vi "Regenerate Hawkeye Files.vi"() -> ()   [LabVIEW 2019, in "HawkeyeToolsMenu.lvlib"]
doc: "GUI to compare LabVIEW code between currently checked out branch with any other branch or any of its commits.\n\n(c) 2024 Soliton Technologies. All rights reserved."
uses:
  HawkeyeToolsMenu.lvlib
  <vilib>/Hampel Software Engineering/Git API/Git API/GIT-api.lvclass
  <vilib>/Hampel Software Engineering/Git API/Git API/GIT-api.lvclass/GIT-api.ctl
  <vilib>/Hampel Software Engineering/Git API/Git API/Controls/GIT-Repository States.ctl
  <vilib>/Hampel Software Engineering/Git API/Git API/Accessors/GIT-Set Working Dir.vi
  <userlib>/_OpenG.lib/file/file.llb/File Exists - Scalar__ogtk.vi
  <userlib>/_OpenG.lib/file/file.llb/Valid Path - Traditional__ogtk.vi
  vi.lib/Hawkeye/Hawkeye.lvlib
panel:
  in  "Tab Control":T1(tab)=enum."Main UI"
  in  "LVLib / LVClass / Sub Folder Path":path
  out "Status Indicator":string
  in  "Check Changed Libraries Only?":bool
  in  "Branch to Compare":string(combo)
  in  "Refresh Current Branch":bool
  out "Current Branch":string="origin/main"
  out "Current Branch Status":string
  in  "Stop":bool
  in  "Repo / Workspace Folder Path":path
  in  "Generate":bool
  # "1. Checkout the branch of interest in your system using any method - Git command line, Desktop Git GUI Clients etc.,\n\n2. Specify the local Repository Path.\n\n3. Verify the current branch, its status and select a branch or commit based on the Compare Mode and click on Compare to display the file changes.\n\n4. Double click on a file to initiate LabVIEW code comparison.\n\n5. Once done with required comparisons, exit the tool by closing the window. The tool cleans up the temporary files added during comparison.\n\n\nNote:\n1. This tool uses LabVIEW's VI Comparison Tool which requires LabVIEW Professional Development System.\n2. It is recommended to not use other Git Clients actively when comparing files using this tool to avoid Git command related errors.\n3. It is recommended to commit all changes (working copy) before using this tool for comparison."
  # "This tool uses git diff command to identify the changes. Hence it is recommended to commit all the changes (working copy) to have them considered for comparison. For code comparison, this tool uses LabVIEW's built in VI Comparison Tool.\n\nExample: Identify changes in current branch when comparing with other branch\n\n---A---B---C---D    <== other branch\n               \\\n                 E---F      <== current branch\n\n1. We will need to identify only the file changes introduced by current branch. E and F commits are those changes in the above example (commits after the common ancestor B).\n2. For the identified file changes compare with the other branch (D) to see how it differs. These differences will be our current branch changelist.\n\nWhy only current branch changes?\nIt is most useful to see how the current branch will modify the files when it is getting merged. Best use case for displaying only current branch changelist will be for Pull Request reviews."
  # "1. Repository Path - Local repository path (the top level folder with '.git' hidden folder in it). Git API will be initialized for this repository.\n\n2. Current Branch - Currently checked out branch. The status of the current branch is also displayed at top right. Click Refresh button to update the current branch if it is changed in the system or received new changes via Git Pull.\n\n3. Compare Mode - Select the type of comparison. You can compare the current branch with another branch or with a particular commit of a selected branch.\n\nIn branch comparison mode, you can enter the branch name for comparison in Branch to Compare. Remote branches usually start with \"origin/\" and local branches do not have \"origin/\" prefix. The branch's recent commit is displayed in Recent Commit and its details in Commit Details for reference. \n\nIn commit comparison mode, the commits available in the branch selected in Select Branch are listed in Commit to Compare. For the commit selected in Commit to Compare, its details will be displayed in the Commit Details. Use Commits to Fetch to limit the number of commits obtained and improve the loading time.\n\n     Note: Git doesn't maintain information on when the branch is created. So, all the commits of the selected branch will be displayed (all the way up to the very first commit after repository creation). Without a limit, it increases loading time.\n\n4. Compare - Identifies the file changes and Current Branch Changelist table shows the list of all files that are different in the current branch compared to the branch/commit selected.\n\n     Note: The other branch/commit in comparison would have introduced its own changes that are not part of current branch. Those changes will not be displayed.\n\n5. Filter LabVIEW VI and Control Files - Filter files except VI and CTL files. These require LabVIEW to compare but project, library and classes are text files that can be easily reviewed in the desktop Git GUI clients or in Pull Request of Git web services.\n\n6. LabVIEW Compare Options - Options to decide what to compare in the code. Set the required options before initiating code compare.\n\n7. Double click on the file you wish to compare. LabVIEW opens the compare window for the file from the current branch and the file from the other branch/commit (file will be suffixed with TEMP). It may take a while if the VI/CTL have lot of dependencies to load. Having the project pre-opened and opening this tool from that instance may reduce the loading time. Note that the file from the other branch/commit in comparison may be missing its dependent files which may not be available in the current branch or deleted in the current branch commits. This will cause the file to be in a broken state but does not affect the comparison. Another reason for the broken state may be due to the parent library/class not recognizing this new file with the suffix but this as well will not affect the comparison.\n\n     Note: The files from other branch/commit are placed at the same location in the current branch so that the LabVIEW can load the dependencies appropriately.\n\n8. Viewed Status (mixed checkbox) - A tick mark appears for every file compared or opened. Use the mixed checkbox (below the Current Branch Changelist) to control status for all files.\n\n     Note: Viewed status is only a visual aid for tracking and does not have any other function other than that.\n\n9. Panel Close - Stops the tools execution after removing all the new files introduced into the current branch (TEMP files)."
  # "This GUI helps identify unexpected dependencies across all libraries in a repository. It also supports branch-to-branch comparison, allowing users to analyze dependency changes between any two branches and validate dependencies only for the modified libraries."
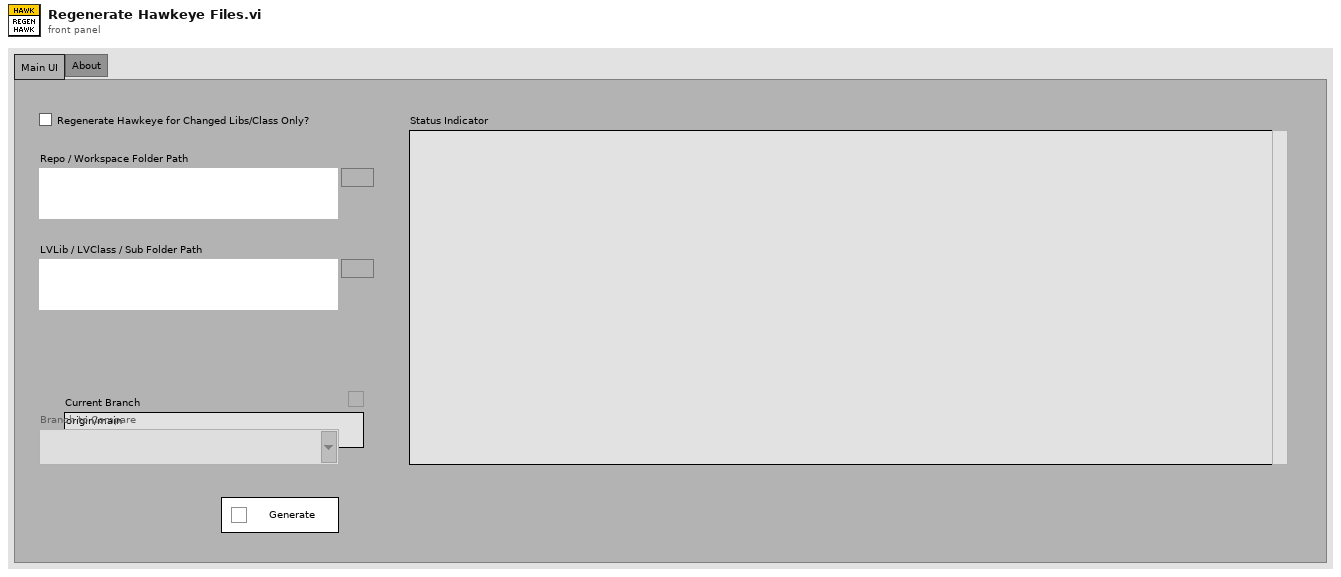
[diagram p1: front panel]
types:
  T1 = enum32{"Getting Started", "How it Works?", "Main UI", "Help", "About"}
  T2 = cluster{"Repository Path":path, "Git API Object":refnum<class "GIT-api.lvclass">, "Git API Initialized?":bool, "Current Branch":string, "Branch to Compare":string, "Check Changed Libraries Only?":bool, "Source Folder Path":path, "Build Specs Folder Path":path}
  T3 = typedef "GIT-API-for-LabVIEW.lvlib/GIT-api.lvclass/GIT-Repository States.ctl" = enum16{"up-to-date", "behind", "ahead", "diverged", "unpublished", "detached", "unknown"}
  T4 = enum8{"Enabled", "Disabled", "Disabled and Grayed Out"}
  T5 = typedef "Hawkeye.lvlib/HawkeyePathConfigs.ctl" = cluster{"GlobalIncludePaths":path[], "GlobalExcludePaths":path[], "BuildSpecsIncludePaths":path[], "ActualDepsIncludePaths":path[], "WorkspacePath":path, "SourceFolderPaths":path[], "ChangedFilesLogpaths":map{string, path}}
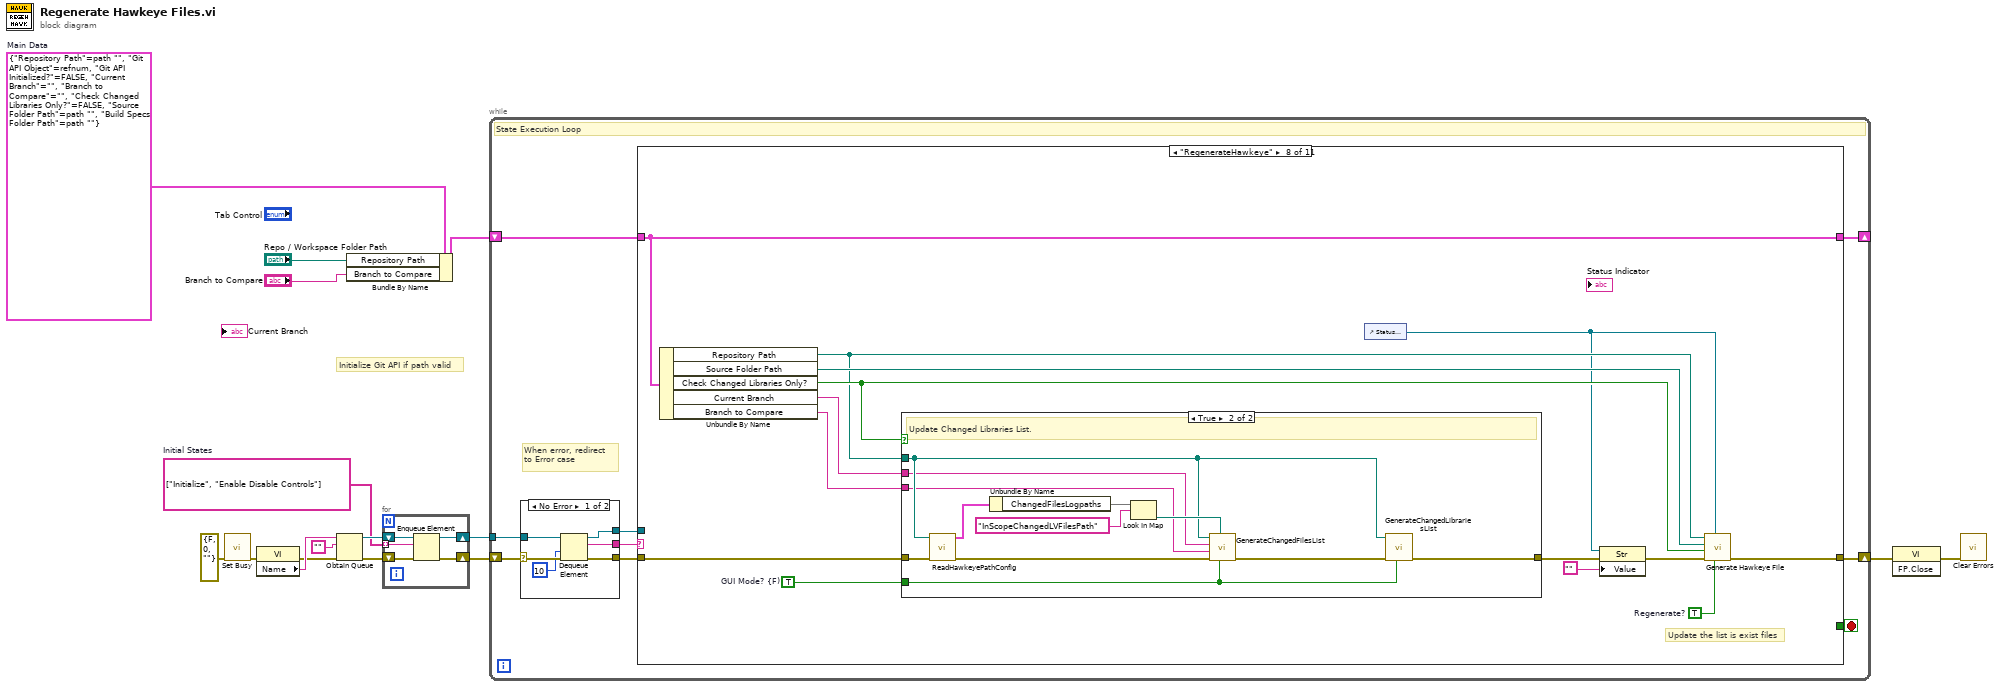
[diagram p0: block diagram]
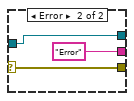
[diagram p2: hidden frame]
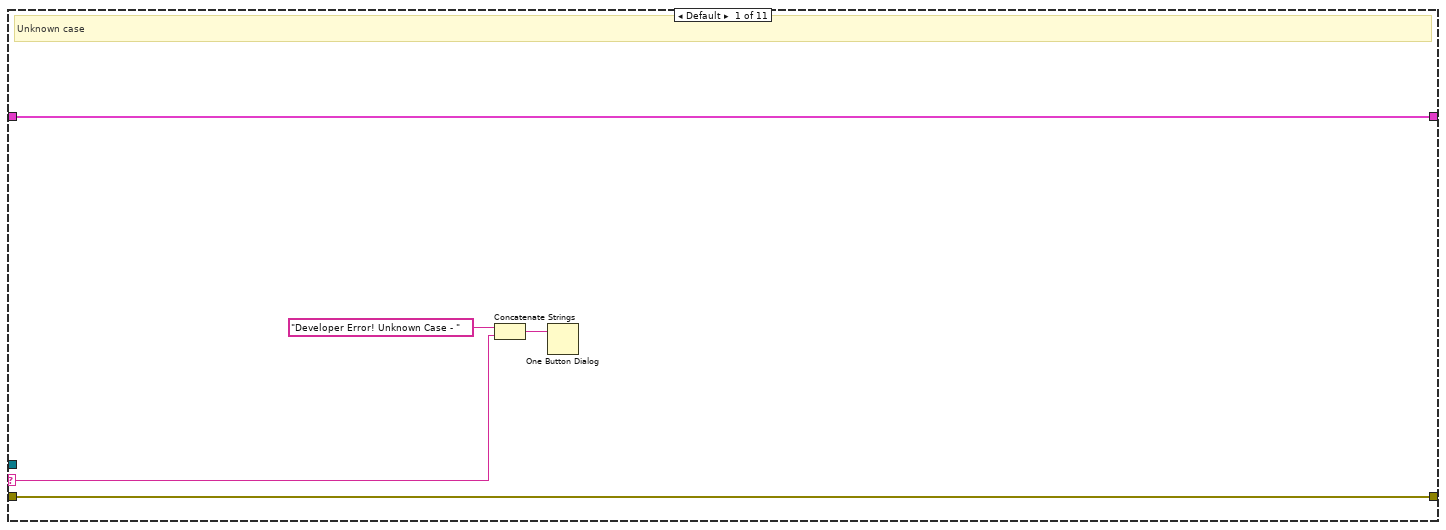
[diagram p3: hidden frame]
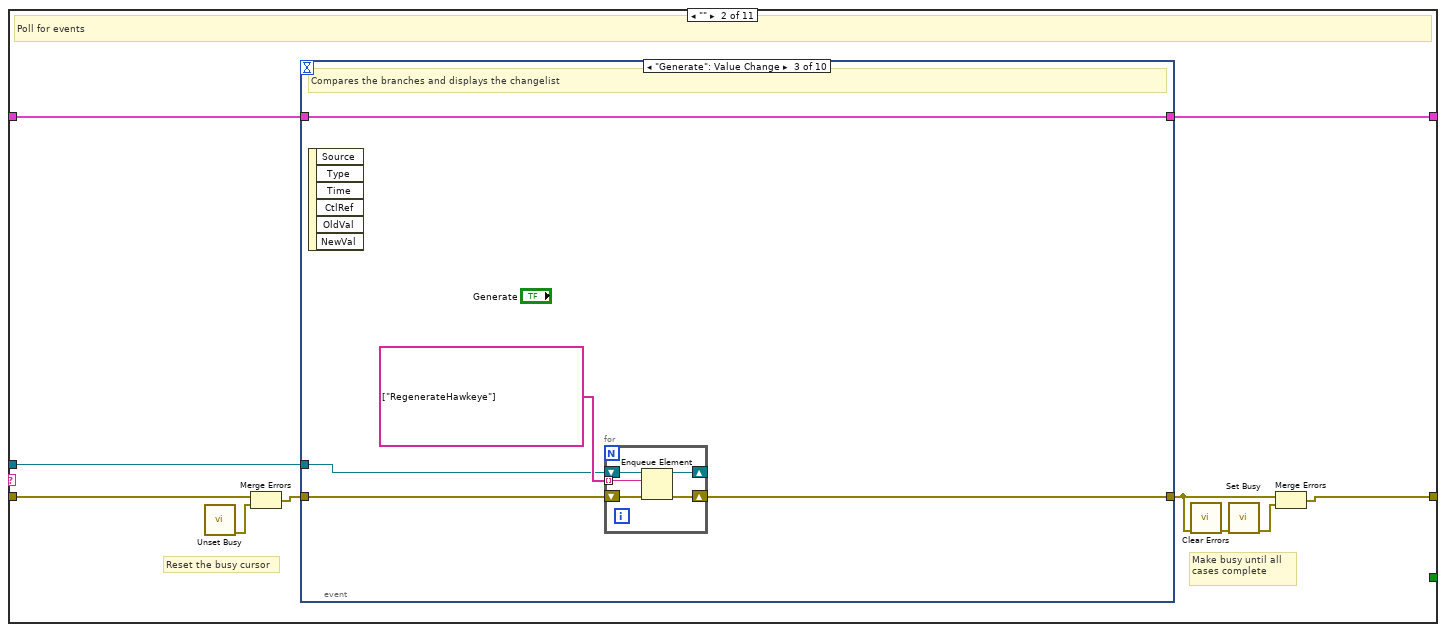
[diagram p4: hidden frame]
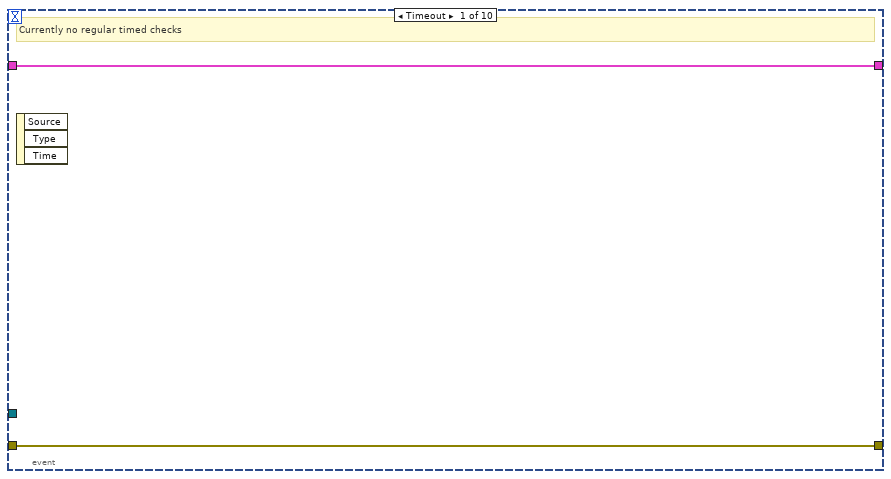
[diagram p5: hidden frame]
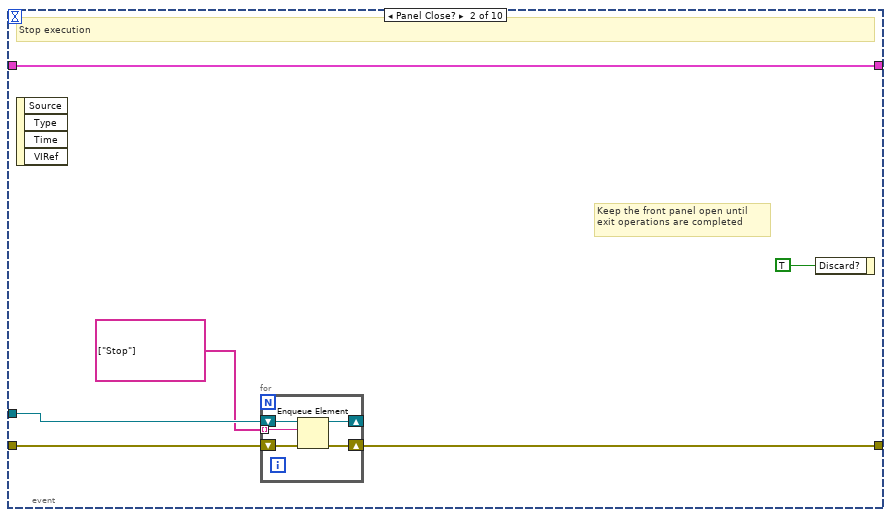
[diagram p6: hidden frame]
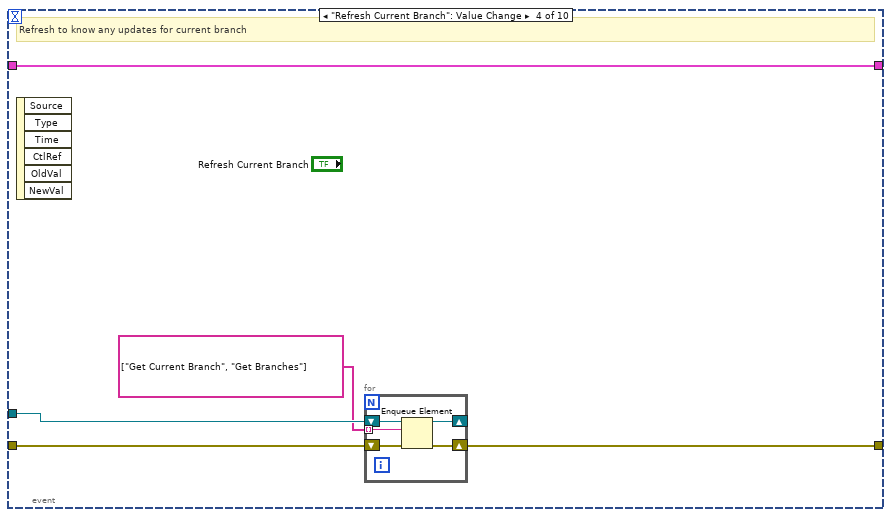
[diagram p7: hidden frame]
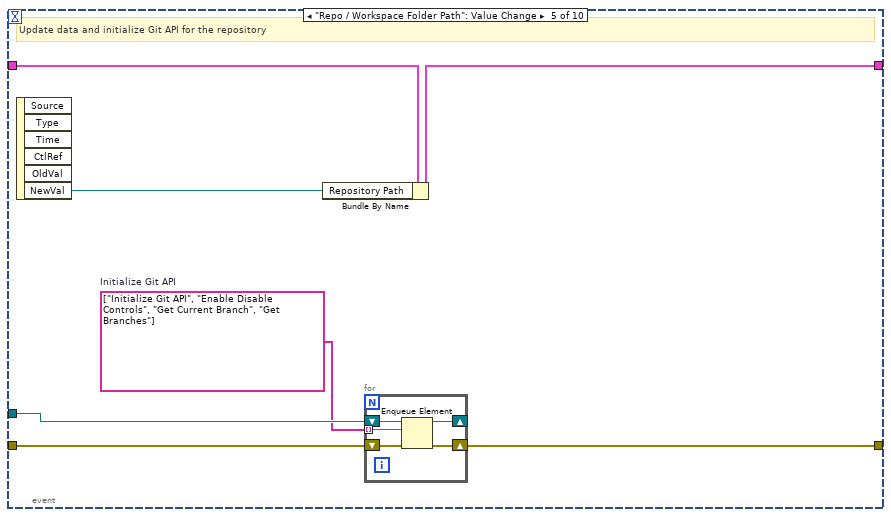
[diagram p8: hidden frame]
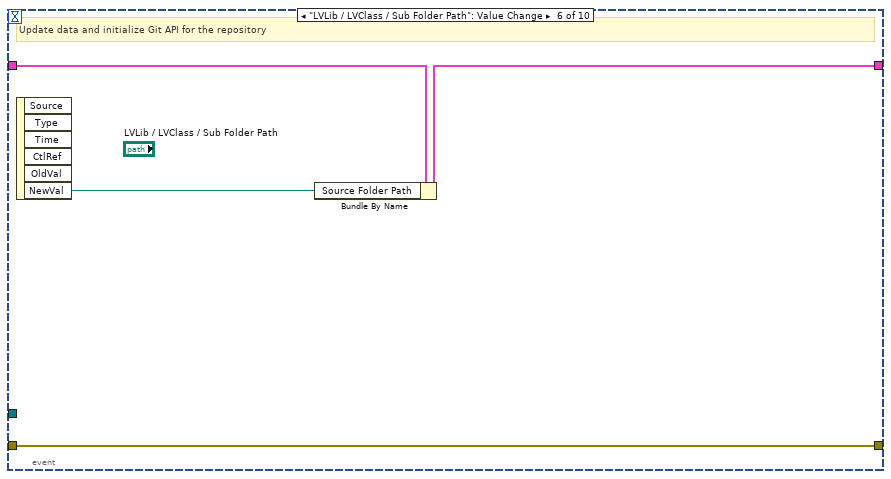
[diagram p9: hidden frame]
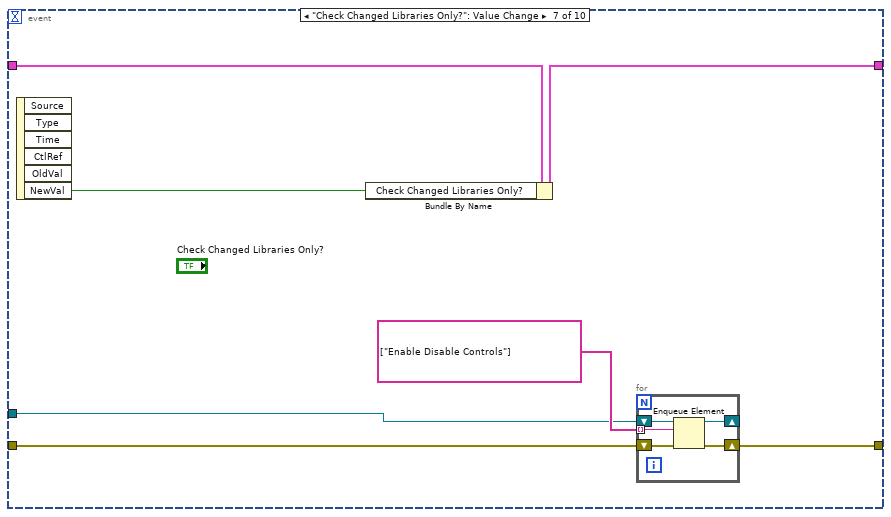
[diagram p10: hidden frame]
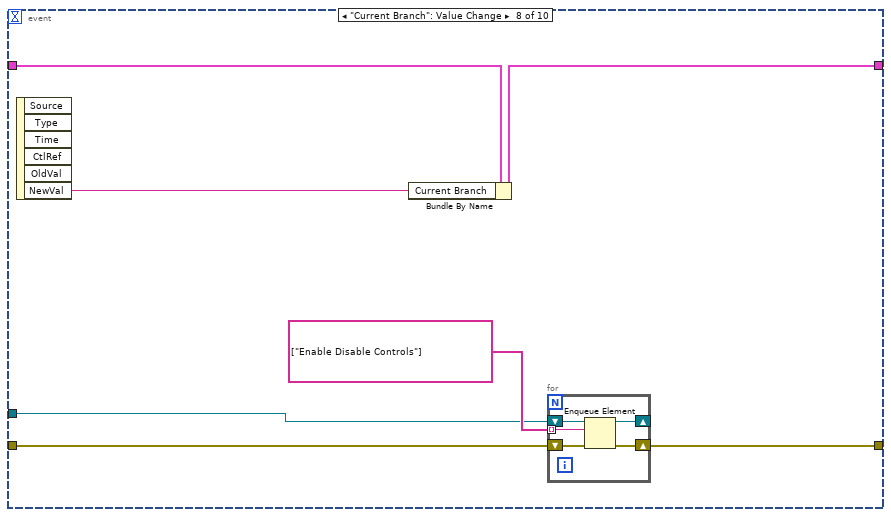
[diagram p11: hidden frame]
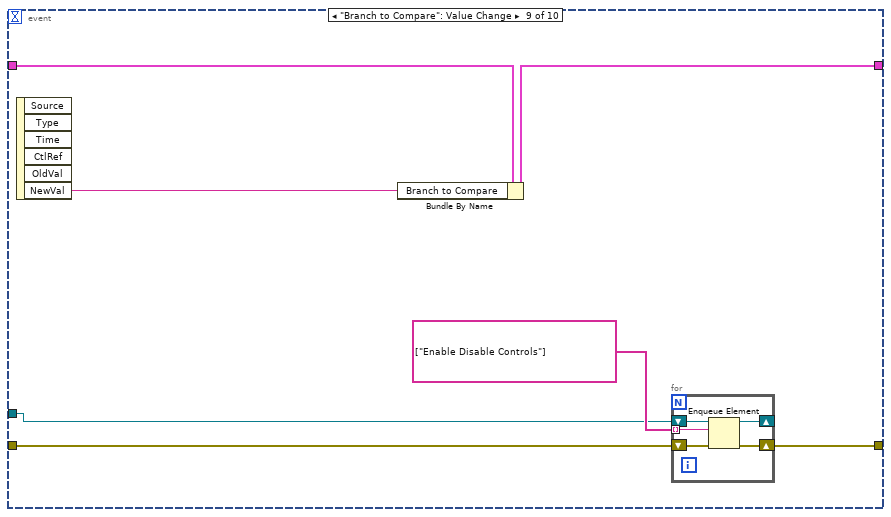
[diagram p12: hidden frame]
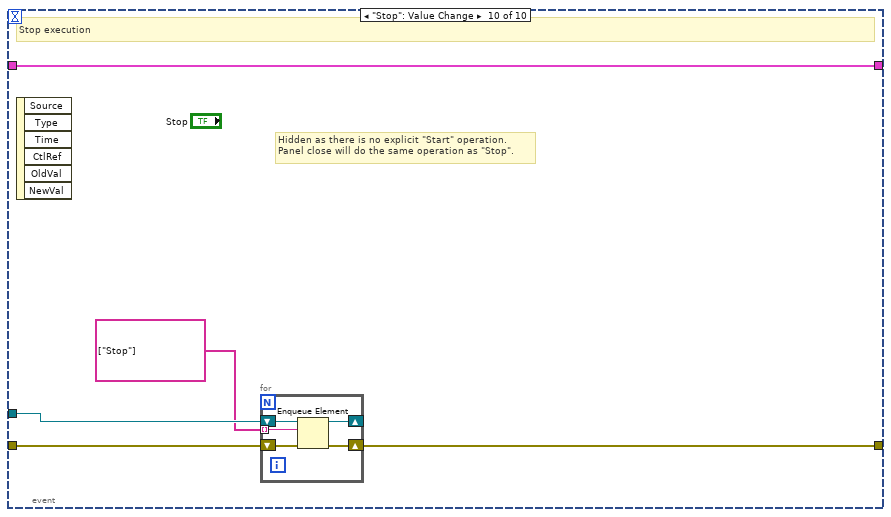
[diagram p13: hidden frame]
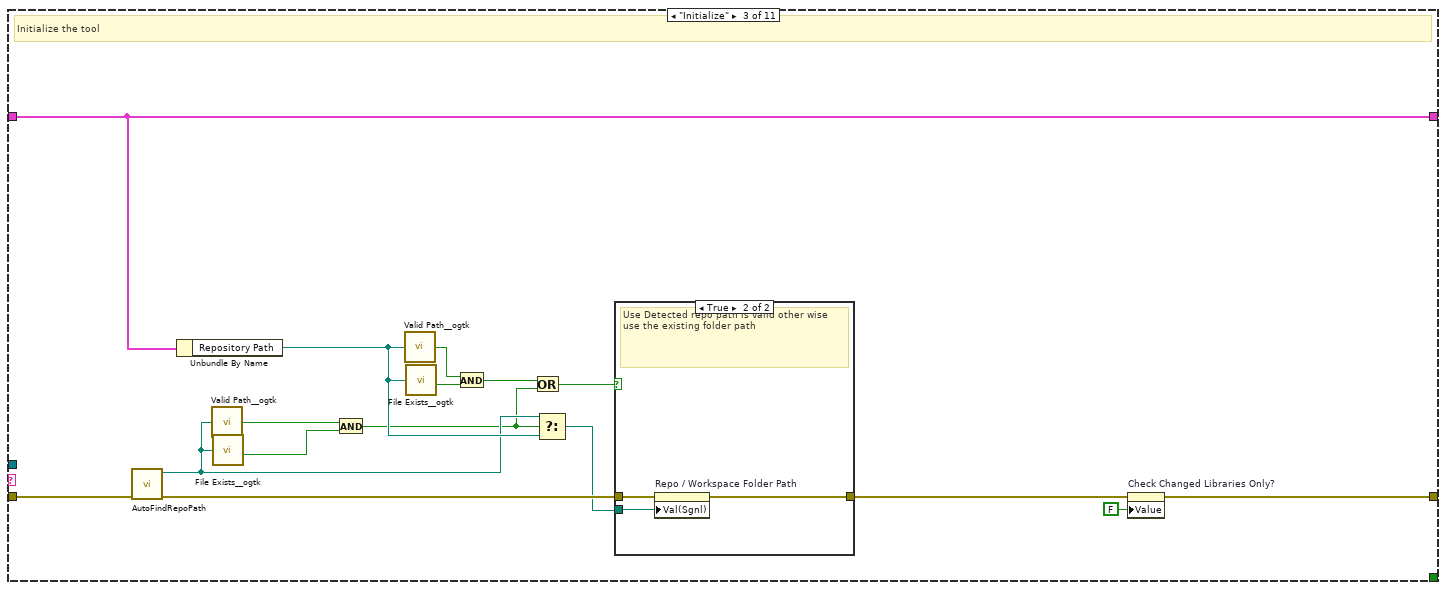
[diagram p14: hidden frame]
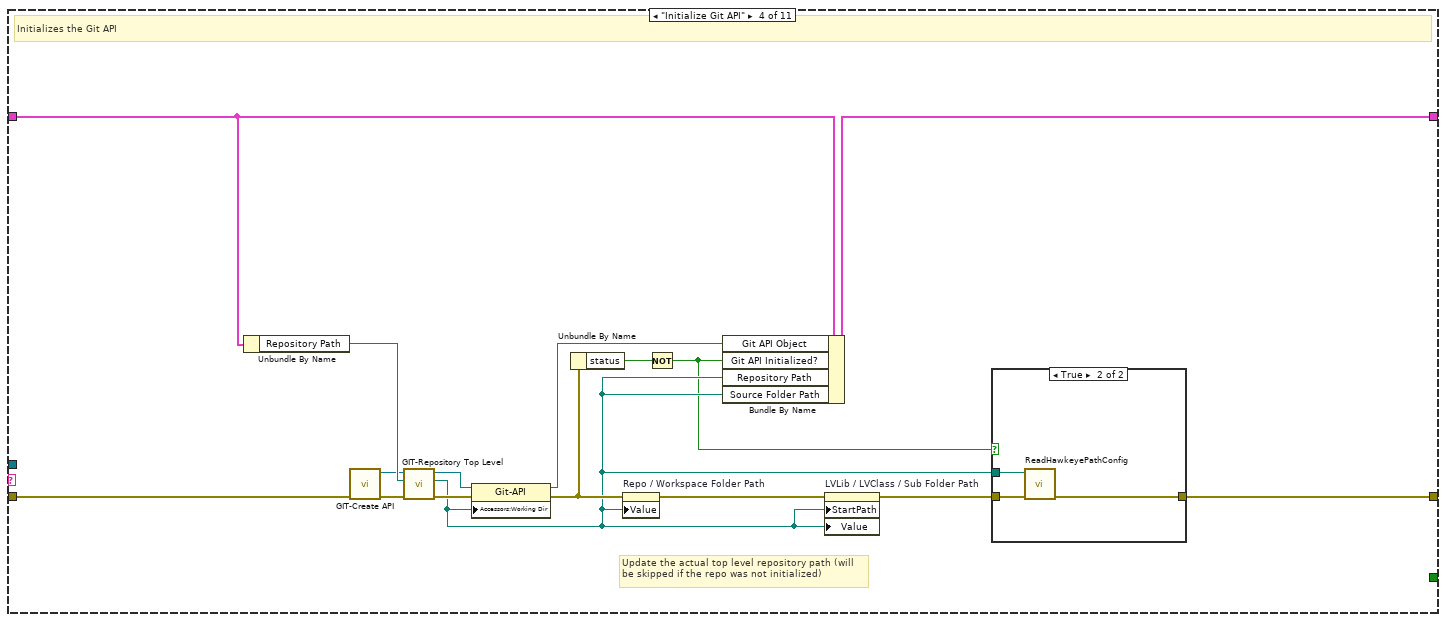
[diagram p16: hidden frame]
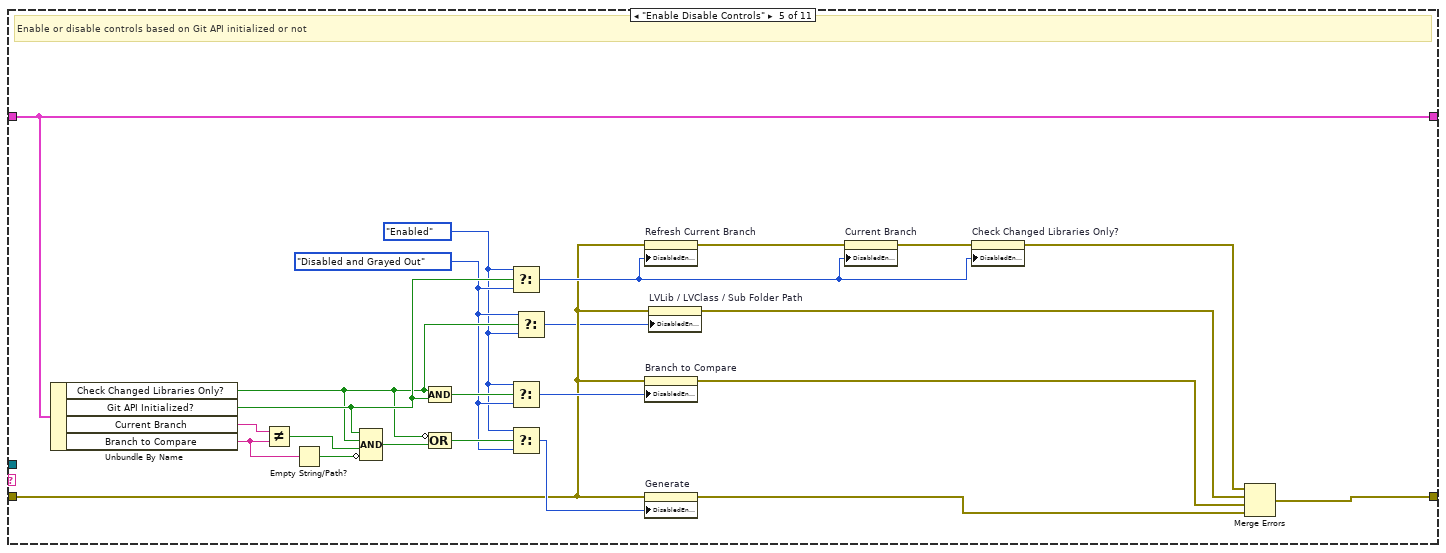
[diagram p18: hidden frame]
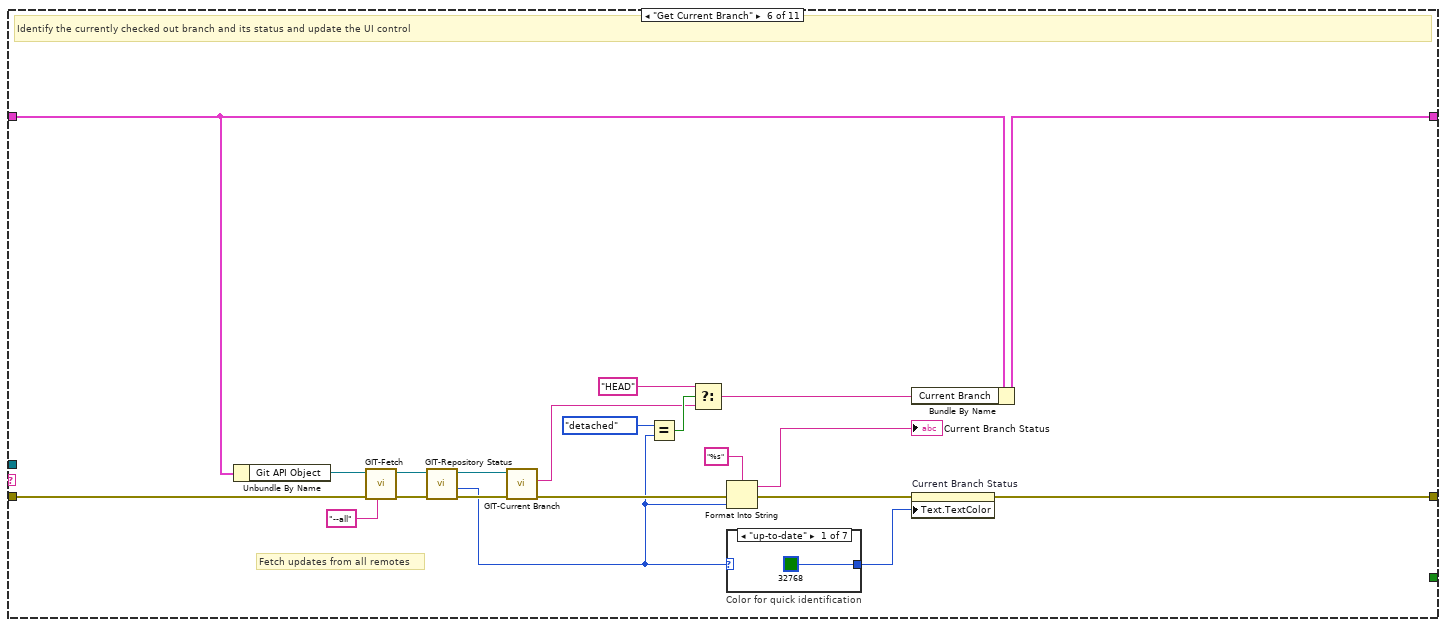
[diagram p19: hidden frame]
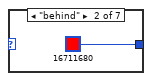
[diagram p20: hidden frame]
diagram:
  w1 = string[] ["Initialize", "Enable Disable Controls"]  # Initial States
  w13 = T2 {"Repository Path"=path "", "Git API Object"=refnum, "Git API Initialized?"=FALSE, "Current Branch"="", "Branch to Compare"="", "Check Changed Libraries Only?"=FALSE, "Source Folder Path"=path "", "Build Specs Folder Path"=path ""}  # Main Data
  # "Initialize Git API if path valid"
  n1 = call <vilib>:"Set Busy.vi"("error in (no error)"=errorcluster {"status"=FALSE, "code"=0, "source"=""}) -> ("error out"=w6:errorcluster)  [unwired: 9 in, 1 out]
  n2 = property class="VI"(error in=w6) -> (error out=w15:errorcluster, "Name"=w16:string)  [unwired: 1 in, 1 out]
  n3 = Obtain Queue(name (unnamed)=w16, element data type="", error in (no error)=w15) -> (queue out=w11:refnum<queue>, error out=w8:errorcluster)  [unwired: 2 in, 1 out]
  n4 = Bundle By Name(cluster=w13, "Repository Path"="Repo / Workspace Folder Path", "Branch to Compare"="Branch to Compare") -> (w12:T2)
  n5 = for {
    tunnel: w1 -> [w18] mode=indexing
    shift-right: [w20] -> w10
    shift-left: w8 -> [w21]
    shift-right: [w17] -> w9
    shift-left: w11 -> [w19]
    n6 = Enqueue Element(queue=w19, element=w18, error in (no error)=w21) -> (queue out=w17:refnum<queue>, error out=w20:errorcluster)  [unwired: 1 in, 1 out]
  }
  n7 = while {
    shift-right: [w22] -> w4
    shift-left: w10 -> [w24]
    tunnel: w9 -> [w25]
    shift-right: [w27] -> _
    shift-left: w12 -> [w26]
    stop <- w28 stop-if-true
    # "When error, redirect to Error case"
    # "State Execution Loop"
    n8 = case shown="No Error" w24 {
      selector: w24 -> [w33 w37]
      tunnel: [w36 "Error" ("element")] -> w30
      tunnel: [w35 w39] -> w29
      tunnel: w25 -> [w34 w39]
      tunnel: [w31 w37] -> w23
      frame No Error {
        n9 = Dequeue Element(queue=w34, timeout in ms (-1)=10, error in (no error)=w33) -> (queue out=w35:refnum<queue>, element=w36:string, error out=w31:errorcluster)  [unwired: 1 out]
      }
      frame Error {
      }
    }
    n10 = case shown="\"RegenerateHawkeye\"" w30 {
      selector: w30 -> [w43 _ _ _ _ _ _ _ _ _ _]
      tunnel: w23 -> [w41 w48 w162 w185 w195 w219 w265 w296 w316 w326 w334]
      tunnel: w29 -> [_ w54 _ _ _ _ _ _ w314 w323 w331]
      tunnel: [w41 w50 w165 w171 w212 w228 w274 w292 w315 w322 w327] -> w22
      tunnel: [_ _ _ _ _ _ _ _ _ w324 _] -> w28
      tunnel: [w40 w52 w159 w182 w213 w231 w272 w297 w313 w325 w335] -> w27
      tunnel: w26 -> [w40 w53 w159 w184 w213 w232 w273 w297 w313 w325 w335]
      frame Default {
        # "Unknown case"
        n11 = Concatenate Strings("Developer Error! Unknown Case - " ("string"), w43) -> (w42:string)
        n12 = One Button Dialog(message=w42) -> ()  [unwired: 1 in, 1 out]
      }
      frame "" {
        # "Reset the busy cursor"
        # "Make busy until all cases complete"
        # "Poll for events"
        n13 = call <vilib>:"Unset Busy.vi"() -> ("error out"=w49:errorcluster)  [unwired: 11 in]
        n14 = Merge Errors(w48, w49) -> (w47:errorcluster)
        n15 = event shown="[2] \"Generate\": Value Change" {
          selector: _ -> [_ _ _ _ _ _ _ _ _ _]
          dyn-events: _ -> [_ _ _ _ _ _ _ _ _ _]
          timeout: _ -> [_ _ _ _ _ _ _ _ _ _]
          tunnel: w47 -> [w55 w62 w71 w82 w91 w100 w105 w116 w128 w144]
          tunnel: w54 -> [_ w61 w70 w81 w90 _ w104 w118 w130 w143]
          tunnel: [w55 w60 w69 w79 w89 w100 w106 w117 w129 w142] -> w46
          tunnel: w53 -> [w56 w59 w68 w78 w94 w103 w110 w122 w134 w141]
          tunnel: [w56 w59 w68 w78 w93 w102 w109 w121 w133 w141] -> w52
          event Timeout {
            # "Currently no regular timed checks"
            n16 = event-data() -> ()  [unwired: 1 in, 3 out]
          }
          event Panel Close? {
            # "Keep the front panel open until exit operations are completed"
            # "Stop execution"
            n17 = event-data() -> ()  [unwired: 1 in, 4 out]
            n18 = for {
              tunnel: string[] ["Stop"] -> [w64] mode=indexing
              shift-right: [w66] -> w60
              shift-left: w62 -> [w67]
              shift-right: [w63] -> _
              shift-left: w61 -> [w65]
              n19 = Enqueue Element(queue=w65, element=w64, error in (no error)=w67) -> (queue out=w63:refnum<queue>, error out=w66:errorcluster)  [unwired: 1 in, 1 out]
            }
            n20 = event-data("Discard?"=TRUE) -> ()  [unwired: 1 in, 1 out]
          }
          event "Generate": Value Change {
            # "Compares the branches and displays the changelist"
            n21 = event-data() -> ()  [unwired: 1 in, 6 out]
            n22 = for {
              tunnel: string[] ["RegenerateHawkeye"] -> [w74] mode=indexing
              shift-right: [w76] -> w69
              shift-left: w71 -> [w77]
              shift-right: [w73] -> _
              shift-left: w70 -> [w75]
              n23 = Enqueue Element(queue=w75, element=w74, error in (no error)=w77) -> (queue out=w73:refnum<queue>, error out=w76:errorcluster)  [unwired: 1 in, 1 out]
            }
          }
          event "Refresh Current Branch": Value Change {
            # "Refresh to know any updates for current branch"
            n24 = event-data() -> ()  [unwired: 1 in, 6 out]
            n25 = for {
              tunnel: string[] ["Get Current Branch", "Get Branches"] -> [w84] mode=indexing
              shift-right: [w86] -> w79
              shift-left: w82 -> [w87]
              shift-right: [w83] -> _
              shift-left: w81 -> [w85]
              n26 = Enqueue Element(queue=w85, element=w84, error in (no error)=w87) -> (queue out=w83:refnum<queue>, error out=w86:errorcluster)  [unwired: 1 in, 1 out]
            }
          }
          event "Repo / Workspace Folder Path": Value Change {
            w88 = string[] ["Initialize Git API", "Enable Disable Controls", "Get Current Branch", "Get Branches"]  # Initialize Git API
            # "Update data and initialize Git API for the repository"
            n27 = event-data() -> ("NewVal"=w92:path)  [unwired: 1 in, 5 out]
            n28 = Bundle By Name(cluster=w94, "Repository Path"=w92) -> (w93:T2)
            n29 = for {
              tunnel: w88 -> [w96] mode=indexing
              shift-right: [w98] -> w89
              shift-left: w91 -> [w99]
              shift-right: [w95] -> _
              shift-left: w90 -> [w97]
              n30 = Enqueue Element(queue=w97, element=w96, error in (no error)=w99) -> (queue out=w95:refnum<queue>, error out=w98:errorcluster)  [unwired: 1 in, 1 out]
            }
          }
          event "LVLib / LVClass / Sub Folder Path": Value Change {
            # "Update data and initialize Git API for the repository"
            n31 = event-data() -> ("NewVal"=w101:path)  [unwired: 1 in, 5 out]
            n32 = Bundle By Name(cluster=w103, "Source Folder Path"=w101) -> (w102:T2)
          }
          event "Check Changed Libraries Only?": Value Change {
            n33 = event-data() -> ("NewVal"=w108:bool)  [unwired: 1 in, 5 out]
            n34 = Bundle By Name(cluster=w110, "Check Changed Libraries Only?"=w108) -> (w109:T2)
            n35 = for {
              tunnel: string[] ["Enable Disable Controls"] -> [w112] mode=indexing
              shift-right: [w114] -> w106
              shift-left: w105 -> [w115]
              shift-right: [w111] -> _
              shift-left: w104 -> [w113]
              n36 = Enqueue Element(queue=w113, element=w112, error in (no error)=w115) -> (queue out=w111:refnum<queue>, error out=w114:errorcluster)  [unwired: 1 in, 1 out]
            }
          }
          event "Current Branch": Value Change {
            n37 = event-data() -> ("NewVal"=w120:string)  [unwired: 1 in, 5 out]
            n38 = Bundle By Name(cluster=w122, "Current Branch"=w120) -> (w121:T2)
            n39 = for {
              tunnel: string[] ["Enable Disable Controls"] -> [w124] mode=indexing
              shift-right: [w126] -> w117
              shift-left: w116 -> [w127]
              shift-right: [w123] -> _
              shift-left: w118 -> [w125]
              n40 = Enqueue Element(queue=w125, element=w124, error in (no error)=w127) -> (queue out=w123:refnum<queue>, error out=w126:errorcluster)  [unwired: 1 in, 1 out]
            }
          }
          event "Branch to Compare": Value Change {
            n41 = event-data() -> ("NewVal"=w132:string)  [unwired: 1 in, 5 out]
            n42 = Bundle By Name(cluster=w134, "Branch to Compare"=w132) -> (w133:T2)
            n43 = for {
              tunnel: string[] ["Enable Disable Controls"] -> [w136] mode=indexing
              shift-right: [w138] -> w129
              shift-left: w128 -> [w139]
              shift-right: [w135] -> _
              shift-left: w130 -> [w137]
              n44 = Enqueue Element(queue=w137, element=w136, error in (no error)=w139) -> (queue out=w135:refnum<queue>, error out=w138:errorcluster)  [unwired: 1 in, 1 out]
            }
          }
          event "Stop": Value Change {
            # "Hidden as there is no explicit \"Start\" operation.\nPanel close will do the same operation as \"Stop\"."
            # "Stop execution"
            n45 = event-data() -> ()  [unwired: 1 in, 6 out]
            n46 = for {
              tunnel: string[] ["Stop"] -> [w146] mode=indexing
              shift-right: [w148] -> w142
              shift-left: w144 -> [w149]
              shift-right: [w145] -> _
              shift-left: w143 -> [w147]
              n47 = Enqueue Element(queue=w147, element=w146, error in (no error)=w149) -> (queue out=w145:refnum<queue>, error out=w148:errorcluster)  [unwired: 1 in, 1 out]
            }
          }
        }
        n48 = call <vilib>:"Clear Errors.vi"("error in (no error)"=w46) -> ("error out"=w45:errorcluster)  [unwired: 5 in, 1 out]
        n49 = call <vilib>:"Set Busy.vi"("error in (no error)"=w45) -> ("error out"=w51:errorcluster)  [unwired: 9 in, 1 out]
        n50 = Merge Errors(w46, w51) -> (w50:errorcluster)
      }
      frame "Initialize" {
        # "Initialize the tool"
        n51 = call "AutoFindRepoPath.vi"("error in (no error)"=w162) -> ("error out"=w163:errorcluster, "Repo Path"=w153:path)  [unwired: 9 in]
        n52 = Unbundle By Name(w159) -> ("Repository Path"=w155:path)
        n53 = call-poly <userlib>:"Valid Path__ogtk.vi"("path"=w153) -> ("valid"=w160:bool)
        n54 = call-poly <userlib>:"File Exists__ogtk.vi"("file path"=w153) -> ("exists"=w161:bool)  [unwired: 6 in, 1 out]
        n55 = And(x=w160, y=w161) -> (x .and. y?=w152:bool)
        n56 = call-poly <userlib>:"Valid Path__ogtk.vi"("path"=w155) -> ("valid"=w154:bool)
        n57 = call-poly <userlib>:"File Exists__ogtk.vi"("file path"=w155) -> ("exists"=w158:bool)  [unwired: 6 in, 1 out]
        n58 = And(x=w154, y=w158) -> (x .and. y?=w157:bool)
        n59 = Or(x=w157, y=w152) -> (x .or. y?=w156:bool)
        n60 = Select(t=w153, s=w152, f=w155) -> (s? t:f=w150:path)
        n61 = case shown="True" w156 {
          tunnel: w163 -> [w166 w169]
          tunnel: [w166 w167] -> w151
          tunnel: w150 -> [_ w168]
          frame False {
          }
          frame True {
            # "Use Detected repo path is valid other wise use the existing folder path"
            n62 = property on="Repo / Workspace Folder Path" class="Path"(error in=w169, "Val(Sgnl)"=w168) -> (error out=w167:errorcluster)  [unwired: 1 in, 1 out]
          }
        }
        n63 = property on="Check Changed Libraries Only?" class="Bool (strict)"(error in=w151, "Value"=FALSE ("Check Changed Libraries Only?")) -> (error out=w165:errorcluster)  [unwired: 1 in, 1 out]
      }
      frame "Initialize Git API" {
        # "Update the actual top level repository path (will be skipped if the repo was not initialized)"
        # "Initializes the Git API"
        n64 = Unbundle By Name(w184) -> ("Repository Path"=w181:path)
        n65 = call <vilib>:"GIT-Create API.vi"("error in"=w185) -> ("error out"=w180:errorcluster, "git-api out"=w178:refnum<class "GIT-api.lvclass">)  [unwired: 9 in]
        n66 = call <vilib>:"GIT-Repository Top Level.vi"("error in"=w180, "Current Path"=w181, "git-api in"=w178) -> ("error out"=w177:errorcluster, "Repo Top Level Path"=w173:path, "git-api out"=w179:refnum<class "GIT-api.lvclass">)  [unwired: 6 in]
        n67 = property class="Git-API"(reference=w179, error in=w177, "Accessors:Working Dir"=w173) -> (reference out=w183:refnum<class "GIT-api.lvclass">, error out=w175:errorcluster)
        n68 = Unbundle By Name(w175) -> ("status"=w176:bool)
        n69 = property on="Repo / Workspace Folder Path" class="Path"(error in=w175, "Value"=w173) -> (error out=w174:errorcluster)  [unwired: 1 in, 1 out]
        n70 = Not(x=w176) -> (.not. x?=w170:bool)
        n71 = Bundle By Name(cluster=w184, "Git API Object"=w183, "Git API Initialized?"=w170, "Repository Path"=w173, "Source Folder Path"=w173) -> (w182:T2)
        n72 = property on="LVLib / LVClass / Sub Folder Path" class="Path"(error in=w174, "StartPath"=w173, "Value"=w173) -> (error out=w172:errorcluster)  [unwired: 1 in, 1 out]
        n73 = case shown="True" w170 {
          tunnel: w173 -> [_ w189]
          tunnel: w172 -> [w186 w188]
          tunnel: [w186 w187] -> w171
          frame False {
          }
          frame True {
            n74 = call "ReadHawkeyePathConfig.vi"("error in (no error)"=w188, "Workspace Path"=w189) -> ("error out"=w187:errorcluster)  [unwired: 8 in, 1 out]
          }
        }
      }
      frame "Enable Disable Controls" {
        w192 = T4."Disabled and Grayed Out" ("Disabled")
        w191 = T4."Enabled" ("Disabled")
        # "Enable or disable controls based on Git API initialized or not"
        n75 = Unbundle By Name(w213) -> ("Check Changed Libraries Only?"=w193:bool, "Git API Initialized?"=w200:bool, "Current Branch"=w208:string, "Branch to Compare"=w204:string)
        n76 = Not Equal?(x=w208, y=w204) -> (x != y?=w201:bool)
        n77 = Empty String/Path?(string/path=w204) -> (empty?=w203:bool)
        n78 = Compound Arithmetic op=AND(w200, w193, w201, invert w203) -> (w202:bool)
        n79 = Compound Arithmetic op=AND(w193, w200) -> (w207:bool)
        n80 = Compound Arithmetic op=OR(invert w193, w202) -> (w209:bool)
        n81 = Select(t=w191, s=w200, f=w192) -> (s? t:f=w196:T4)
        n82 = Select(t=w191, s=w207, f=w192) -> (s? t:f=w206:T4)
        n83 = Select(t=w191, s=w209, f=w192) -> (s? t:f=w210:T4)
        n84 = Select(t=w192, s=w193, f=w191) -> (s? t:f=w190:T4)
        n85 = property on="Refresh Current Branch" class="Bool"(error in=w195, "DisabledEnum"=w196) -> (error out=w199:errorcluster)  [unwired: 1 in, 1 out]
        n86 = property on="Branch to Compare" class="CmbBox"(error in=w195, "DisabledEnum"=w206) -> (error out=w211:errorcluster)  [unwired: 1 in, 1 out]
        n87 = property on="Generate" class="Bool"(error in=w195, "DisabledEnum"=w210) -> (error out=w205:errorcluster)  [unwired: 1 in, 1 out]
        n88 = property on="LVLib / LVClass / Sub Folder Path" class="Path"(error in=w195, "DisabledEnum"=w190) -> (error out=w194:errorcluster)  [unwired: 1 in, 1 out]
        n89 = property on="Current Branch" class="Str"(error in=w199, "DisabledEnum"=w196) -> (error out=w198:errorcluster)  [unwired: 1 in, 1 out]
        n90 = property on="Check Changed Libraries Only?" class="Bool (strict)"(error in=w198, "DisabledEnum"=w196) -> (error out=w197:errorcluster)  [unwired: 1 in, 1 out]
        n91 = Merge Errors(w197, w194, w211, w205) -> (w212:errorcluster)
      }
      frame "Get Current Branch" {
        # "Fetch updates from all remotes"
        # "Identify the currently checked out branch and its status and update the UI control"
        n92 = Unbundle By Name(w232) -> ("Git API Object"=w220:refnum<class "GIT-api.lvclass">)
        n93 = call <vilib>:"GIT-Fetch.vi"("param"="--all", "error in"=w219, "git-api in"=w220) -> ("error out"=w225:errorcluster, "git-api out"=w226:refnum<class "GIT-api.lvclass">)  [unwired: 6 in, 1 out]
        n94 = call <vilib>:"GIT-Repository Status.vi"("error in"=w225, "git-api in"=w226) -> ("error out"=w234:errorcluster, "State"=w217:T3, "git-api out"=w233:refnum<class "GIT-api.lvclass">)  [unwired: 6 in, 1 out]
        n95 = call <vilib>:"GIT-Current Branch.vi"("error in"=w234, "git-api in"=w233) -> ("error out"=w218:errorcluster, "current branch"=w221:string)  [unwired: 7 in, 1 out]
        n96 = Equal?(x=GIT-Repository_States."detached", y=w217) -> (x = y?=w222:bool)
        n97 = Select(t="HEAD", s=w222, f=w221) -> (s? t:f=w214:string)
        n98 = Format Into String(format string="%s", error in=w218, w217) -> (resulting string=→"Current Branch Status":string, error out=w215:errorcluster)  [unwired: 1 in]
        n99 = case "Color for quick identification" shown="\"up-to-date\"" w217 {
          tunnel: [u32 32768 u32 16711680 u32 16860 u32 16744448 u32 16777222 u32 7171459 u32 16711680] -> w227
          frame "up-to-date" {
          }
          frame "behind" {
          }
          frame "ahead" {
          }
          frame "diverged" {
          }
          frame "unpublished" {
          }
          frame "detached" {
          }
          frame "unknown" {
          }
        }
        n100 = Bundle By Name(cluster=w232, "Current Branch"=w214) -> (w231:T2)
        n101 = property on="Current Branch Status" class="Str"(error in=w215, "Text.TextColor"=w227) -> (error out=w228:errorcluster)  [unwired: 1 in, 1 out]
      }
      frame "Get Branches" {
        w255 = 0  # Branch Name List
        w260 = string[][] []
        w259 = "%s" ("format string")
        # "Reset if previous value not found"
        # "Combine local and remote branches"
        # "List Local branches"
        # "List Remote branches\nNote: All remote branches usually start with origin/ unless renamed"
        # "Reset if previous value not found"
        # "Get all local and remote branches and update UI control"
        n102 = Unbundle By Name(w273) -> ("Current Branch"=w245:string, "Git API Object"=w263:refnum<class "GIT-api.lvclass">)
        n103 = call <vilib>:"GIT-Branch.vi"("error in"=w265, "git-api in"=w263) -> ("error out"=w264:errorcluster, "std out"=w256:string, "git-api out"=w257:refnum<class "GIT-api.lvclass">)  [unwired: 7 in]
        n104 = call <vilib>:"GIT-Branch.vi"("param"="-r", "error in"=w264, "git-api in"=w257) -> ("error out"=w267:errorcluster, "std out"=w258:string)  [unwired: 6 in, 1 out]
        n105 = Spreadsheet String To Array(format string=w259, spreadsheet string=w256, array type (2D Dbl)=w260) -> (array=w275:string[][])  [unwired: 1 in]
        n106 = Spreadsheet String To Array(format string=w259, spreadsheet string=w258, array type (2D Dbl)=w260) -> (array=w261:string[][])  [unwired: 1 in]
        n107 = Index Array(array=w275, index (col)=w255) -> (element=w262:string[])  [unwired: 1 in]
        n108 = Index Array(array=w261, index (col)=w255) -> (element=w251:string[])  [unwired: 1 in]
        n109 = for "Remove current branch pointer" {
          tunnel: w262 -> [w284] mode=indexing
          tunnel: [w280] -> w254 mode=indexing
          tunnel: [w279] -> w276 mode=indexing
          n110 = Search and Replace String(input string=w284, search string="*", replace string="") -> (result string=w281:string, error out=w279:errorcluster)  [unwired: 5 in, 2 out]
          n111 = call <vilib>:"Trim Whitespace.vi"("string"=w281) -> ("trimmed string"=w280:string)  [unwired: 1 in]
        }
        n112 = for {
          tunnel: [w278] -> w252 mode=indexing
          tunnel: w251 -> [w277] mode=indexing
          n113 = call <vilib>:"Trim Whitespace.vi"("string"=w277) -> ("trimmed string"=w278:string)  [unwired: 1 in]
        }
        n114 = Build Array (concatenate)(w254, w252) -> (w246:string[])
        n115 = Merge Errors(w267, w276) -> (w253:errorcluster)
        n116 = Search 1D Array(1D array=w246, element=w245) -> (index of element=w248:i32)  [unwired: 1 in]
        n117 = Greater Or Equal To 0?(x=w248) -> (x >= 0?=w249:bool)
        n118 = Select(t=w245, s=w249, f="") -> (s? t:f=w247:string)
        n119 = property on="Current Branch" class="Str"(error in=w253, "Value"=w247) -> (error out=w244:errorcluster)  [unwired: 1 in, 1 out]
        n120 = property on="Branch to Compare" class="CmbBox"(error in=w244, "Strings[]"=w246) -> (error out=w243:errorcluster, "Value"=w242:string)  [unwired: 1 in, 1 out]
        n121 = Search 1D Array(1D array=w246, element=w242) -> (index of element=w271:i32)  [unwired: 1 in]
        n122 = Greater Or Equal To 0?(x=w271) -> (x >= 0?=w270:bool)
        n123 = Select(t=w242, s=w270, f="") -> (s? t:f=w268:string)
        n124 = Bundle By Name(cluster=w273, "Branch to Compare"=w268) -> (w272:T2)
        n125 = property on="Branch to Compare" class="CmbBox"(error in=w243, "Value"=w268) -> (error out=w274:errorcluster)  [unwired: 1 in, 1 out]
      }
      frame "RegenerateHawkeye" {
        w290 = TRUE  # Regenerate?
        w298 = TRUE  # GUI Mode? {F)
        # "Update the list is exist files"
        n126 = Unbundle By Name(w297) -> ("Repository Path"=w288:path, "Source Folder Path"=w289:path, "Check Changed Libraries Only?"=w291:bool, "Current Branch"=w295:string, "Branch to Compare"=w294:string)
        n127 = case shown="True" w291 {
          tunnel: [w299 w310] -> w293
          tunnel: w298 -> [_ w309]
          tunnel: w288 -> [_ w304]
          tunnel: w296 -> [w299 w303]
          tunnel: w295 -> [_ w301]
          tunnel: w294 -> [_ w300]
          frame False {
          }
          frame True {
            # "Update Changed Libraries List."
            n128 = call "ReadHawkeyePathConfig.vi"("error in (no error)"=w303, "Workspace Path"=w304) -> ("error out"=w302:errorcluster, "Hawkeye Path Config Out"=w308:T5)  [unwired: 8 in]
            n129 = Unbundle By Name(w308) -> ("ChangedFilesLogpaths"=w306:map{string, path})
            n130 = Look In Map(map=w306, key="InScopeChangedLVFilesPath") -> (value=w305:path)  [unwired: 1 in, 1 out]
            n131 = call "GenerateChangedFilesList.vi"("GUI Mode? {F)"=w309, "Output File Path"=w305, "error in (no error)"=w302, "Branch 2"=w300, "Branch 1"=w301, "Workspace Path"=w304) -> ("error out"=w311:errorcluster)  [unwired: 5 in]
            n132 = call "GenerateChangedLibrariesList.vi"("GUI Mode? {F)"=w309, "error in (no error)"=w311, "Workspace Path"=w304) -> ("error out"=w310:errorcluster)  [unwired: 8 in]
          }
        }
        n133 = control-ref of="Status Indicator"() -> (w286:refnum<vi>)
        n134 = property class="Str"(reference=w286, error in=w293, "Value"="") -> (error out=w287:errorcluster)  [unwired: 1 out]
        n135 = call "Generate Hawkeye File.vi"("Regenerate?"=w290, "Status Indicator Ref"=w286, "error in (no error)"=w287, "Check Changed Libraries Only?"=w291, "LVLib / LVClass / Sub Folder Path"=w289, "Repo Folder Path"=w288) -> ("error out"=w292:errorcluster)  [unwired: 5 in]
      }
      frame "Stop" {
        # "Performs actions when the VI is stopped."
        n136 = for {
          tunnel: string[] ["Exit"] -> [w318] mode=indexing
          shift-right: [w320] -> w315
          shift-left: w316 -> [w321]
          shift-right: [w317] -> _
          shift-left: w314 -> [w319]
          n137 = Enqueue Element(queue=w319, element=w318, error in (no error)=w321) -> (queue out=w317:refnum<queue>, error out=w320:errorcluster)  [unwired: 1 in, 1 out]
        }
      }
      frame "Exit" {
        w324 = TRUE  # Exit?
        # "Finish the execution"
        n138 = Release Queue(queue=w323, error in (no error)=w326) -> (error out=w322:errorcluster)  [unwired: 1 in, 2 out]
      }
      frame "Error" {
        # "In case of any Git API initialization errors, we need to disable the controls."
        # "Show the error dialog and clear out the operations. Update controls status."
        n139 = call <vilib>:"Simple Error Handler.vi"("error in (no error)"=w334) -> ("error out"=w333:errorcluster)  [unwired: 4 in, 4 out]
        n140 = call <vilib>:"Clear Errors.vi"("error in (no error)"=w333) -> ("error out"=w332:errorcluster)  [unwired: 5 in, 1 out]
        n141 = Flush Queue(queue=w331, error in (no error)=w332) -> (queue out=w328:refnum<queue>, error out=w329:errorcluster)  [unwired: 1 out]
        n142 = for {
          tunnel: string[] ["Enable Disable Controls"] -> [w337] mode=indexing
          shift-right: [w339] -> w327
          shift-left: w329 -> [w340]
          shift-right: [w336] -> _
          shift-left: w328 -> [w338]
          n143 = Enqueue Element(queue=w338, element=w337, error in (no error)=w340) -> (queue out=w336:refnum<queue>, error out=w339:errorcluster)  [unwired: 1 in, 1 out]
        }
      }
    }
  }
  n144 = invoke class="VI" method="FP.Close"(error in=w4) -> (error out=w3:errorcluster)  [unwired: 2 in, 2 out]
  n145 = call <vilib>:"Clear Errors.vi"("error in (no error)"=w3) -> ()  [unwired: 5 in, 2 out]
